vi "TWM Client Recieve Packet.vi"(6 "max message length (1024)":i32=1024, 7 "end of packet key":string="TWM:command:EndOfPacket", 8 "error in":errorcluster, 9 "timeout [ms] (5000 ms)":i32=5000, 10 "message header (empty)":string, 11 "handle in":i32=-1) -> (0 "error out":errorcluster, 2 "message data":string, 3 "handle out":i32)   [LabVIEW 2020, in "TWM Client.lvlib"]
doc: "Receives message from TWM server with timeout. Message is terminated by given key. If header string is passed, the function will check the match with data packet and eventually throw an error."
uses:
  TWM Client.lvlib
  <vilib>/Utility/error.llb/Error Cluster From Error Code.vi
  <vilib>/ErrorRing/Error Ring.xnode
  infolib.lvlib
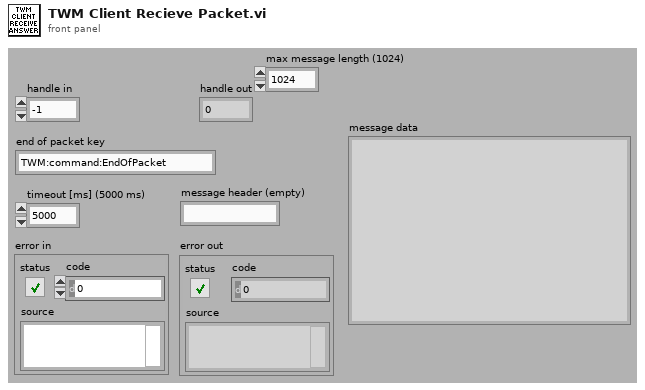
[diagram p1: front panel]
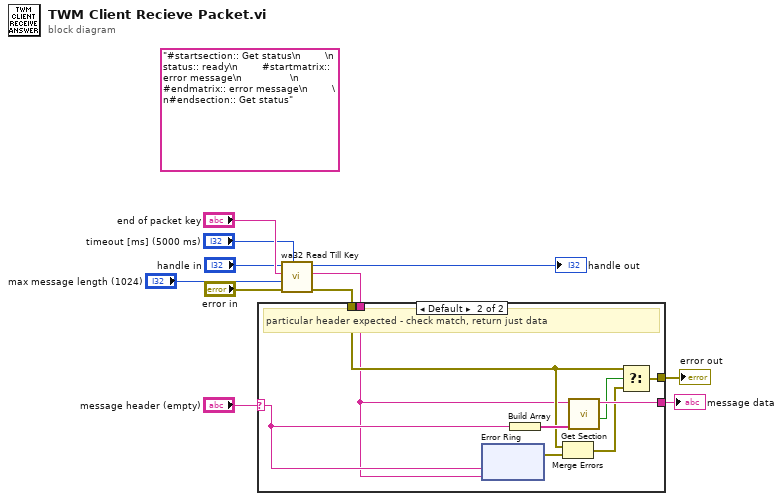
[diagram p0: block diagram]
diagram:
  (unwired) "#startsection:: Get status\n        \n        status:: ready\n        #startmatrix:: error message\n                \n        #endmatrix:: error message\n        \n#endsection:: Get status" ("read message")
  n1 = call "wa32 Read Till Key.vi"("timeout [ms] (1000)"="timeout [ms] (5000 ms)", "error in"="error in", "max message length (1024)"="max message length (1024)", "key string"="end of packet key", "handle"="handle in") -> ("error out"=w2:errorcluster, "read message"=w1:string, "handle out"=→"handle out":i32)  [unwired: 4 in]
  n2 = case shown="Default" "message header (empty)" {
    selector: "message header (empty)" -> [_ w16]
    tunnel: w2 -> [w12 w15]
    tunnel: w1 -> [w13 w14]
    tunnel: [w13 w22] -> w4
    tunnel: [w12 w18] -> w5
    frame "" {
      # "no header expected - retorn everything"
    }
    frame Default {
      # "particular header expected - check match, return just data"
      n3 = xnode "Error Ring"("parameter 0"=w16, "parameter 1"=w14) -> ("error out"=w20:errorcluster)
      n4 = Build Array(w16) -> (w17:string[])
      n5 = Merge Errors(w15, w20) -> (w19:errorcluster)
      n6 = call "Get Section.vi"("sections"=w17, "info data"=w14) -> ("exist"=w21:bool, "section part"=w22:string)  [unwired: 7 in, 1 out]
      n7 = Select(t=w15, s=w21, f=w19) -> (s? t:f=w18:errorcluster)
    }
  }
  "error out" <- w5
  "message data" <- w4
